vi "meTEC_Open Session.vi"(8 "error in (no error)":errorcluster, 11 "COM Port":refnum<visa-resource-name>="COM1") -> (0 "error out":errorcluster, 3 "VISA resource name_OUT":refnum<visa-resource-name>)   [LabVIEW 2019]
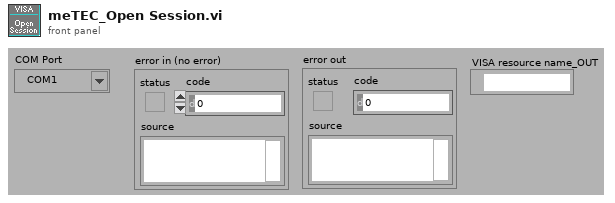
[diagram p1: front panel]
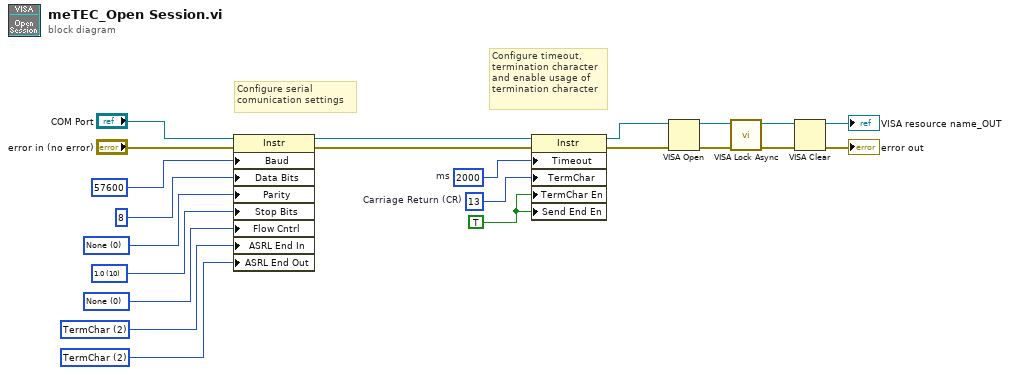
[diagram p0: block diagram]
diagram:
  w6 = u16 2 items=["None", "Last Bit", "TermChar", "Break"] ("Serial Settings:End Mode for Writes")
  w7 = TRUE ("Message Based Settings:Termination Character Enable")
  w16 = u8 13  # Carriage Return (CR)
  w17 = u32 2000  # ms
  w18 = u16 2 items=["None", "Last Bit", "TermChar"] ("Serial Settings:End Mode for Reads")
  w19 = u16 0 items=["None", "XON/XOFF", "RTS/CTS", "XON/XOFF & RTS/CTS", "DTR/DSR", "XON/XOFF & DTR/DSR"] ("Serial Settings:Flow Control")
  w20 = u16 10 items=["1.0"=10, "1.5"=15, "2.0"=20] ("Serial Settings:Stop Bits")
  w21 = u16 0 items=["None", "Odd", "Even", "Mark", "Space"] ("Serial Settings:Parity")
  # "Configure timeout,\ntermination character\nand enable usage of\ntermination character"
  # "Configure serial\ncomunication settings"
  n1 = property class="Instr"(reference="COM Port", error in="error in (no error)", "Baud"=u32 57600 ("Serial Settings:Baud Rate"), "Data Bits"=u16 8 ("Serial Settings:Data Bits"), "Parity"=w21, "Stop Bits"=w20, "Flow Cntrl"=w19, "ASRL End In"=w18, "ASRL End Out"=w6) -> (reference out=w4:refnum<visa-resource-name>, error out=w5:errorcluster)
  n2 = property class="Instr"(reference=w4, error in=w5, "Timeout"=w17, "TermChar"=w16, "TermChar En"=w7, "Send End En"=w7) -> (reference out=w13:refnum<visa-resource-name>, error out=w12:errorcluster)
  n3 = VISA Open(error in (no error)=w12, VISA resource name=w13) -> (VISA resource name=w2:refnum<visa-resource-name>, error out=w11:errorcluster)  [unwired: 3 in]
  n4 = call <vilib>:"VISA Lock Async.vi"("error in (no error)"=w11, "VISA resource name"=w2) -> ("error out"=w3:errorcluster, "VISA resource name out"=w1:refnum<visa-resource-name>)  [unwired: 7 in, 1 out]
  n5 = VISA Clear(VISA resource name=w1, error in (no error)=w3) -> (VISA resource name out=→"VISA resource name_OUT":refnum<visa-resource-name>, error out=→"error out":errorcluster)
